vi "ajouterdonneeprojet.vi"(0 "Deadline":string caption="heure", 1 "Budget":dbl, 2 "Name":string, 3 "Fichier DB":string) -> ()   [LabVIEW 2024]
uses:
  <vilib>/drjdpowell/SQLite Library/SQL Connection/Open (string).vi
  <vilib>/drjdpowell/SQLite Library/SQL Connection/Execute SQL (No results).vi
  <vilib>/drjdpowell/SQLite Library/SQL Connection/Connection.lvclass
  <vilib>/drjdpowell/SQLite Library/SQLite.lvlib
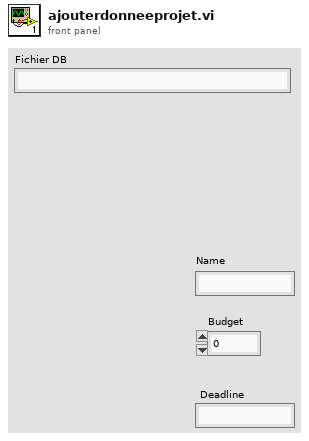
[diagram p1: front panel]
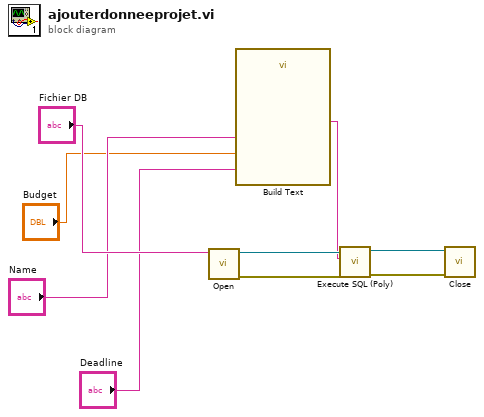
[diagram p0: block diagram]
diagram:
  n1 = call-poly <vilib>:"Open.vi"("db file"="Fichier DB") -> ("error out"=w8:errorcluster, "SQLite Connection"=w9:refnum<class "Connection.lvclass">)  [unwired: 9 in]
  n2 = call "Build Text"("name"="Name", "budget"="Budget", "deadline"="Deadline") -> ("Result"=w7:string)  [unwired: 11 in, 1 out]
  n3 = call-poly <vilib>:"Execute SQL (Poly).vi"("error in (no error)"=w8, "SQL"=w7, "SQLite Connection in"=w9) -> ("error out"=w6:errorcluster, "SQLite Connection"=w5:refnum<class "Connection.lvclass">)  [unwired: 7 in]
  n4 = call-dynamic "Close.vi"("error in (no error)"=w6, "SQLite Connection in"=w5) -> ()  [unwired: 9 in, 1 out]
